vi "SS Class Init.vi"(7 "VI Refnum":refnum<vi>, 8 "error in (no error)":errorcluster, 9 "Init Data":variant, 10 "Device":string, 11 "Subsystem Class Temp Control in":refnum<class "Subsystem Class Temp Control.lvclass">) -> (0 "error out":errorcluster, 2 "Channel List":refnum<class "HK Item.lvclass">[](array[class]), 3 "Subsystem Class Temp Control out":refnum<class "Subsystem Class Temp Control.lvclass">)   [LabVIEW 2022 SP3, in "Subsystem Class Temp Control.lvclass"]
uses:
  Subsystem Class Temp Control.lvclass
  hk-channel-class/hk-channel-class/HK Item/HK Item.lvclass
  Subsystem Class.lvclass
  Subsystem Class Temp Control.lvclass/Subsystem Class Temp Control.ctl
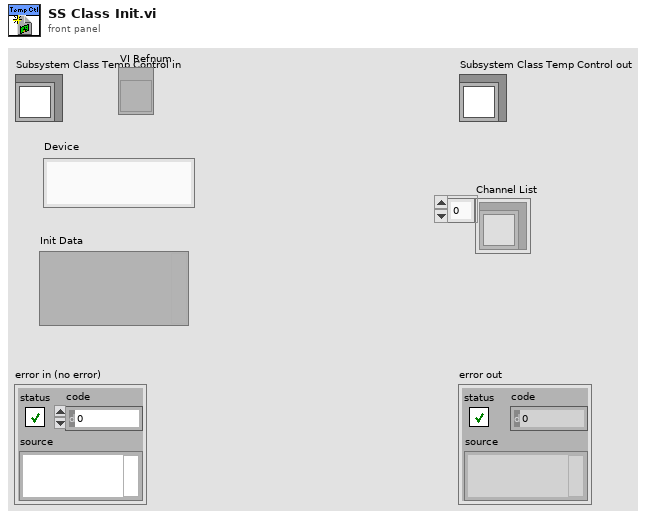
[diagram p1: front panel]
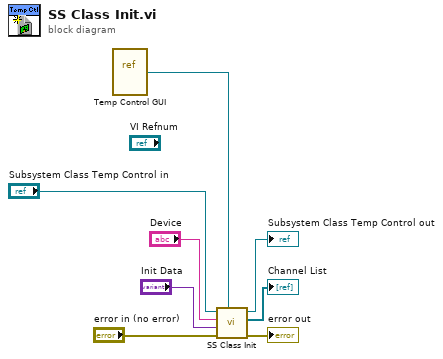
[diagram p0: block diagram]
diagram:
  n1 = vi-ref "Temp Control GUI.vi"() -> (w1:refnum<vi>)
  n2 = call-parent "SS Class Init.vi"("VI Refnum"=w1, "error in (no error)"="error in (no error)", "Init Data"="Init Data", "Device"="Device", "Subsystem Class in"="Subsystem Class Temp Control in") -> ("error out"=→"error out":errorcluster, "Channel List"=→"Channel List":refnum<class "HK Item.lvclass">[], "Subsystem Class out"=→"Subsystem Class Temp Control out":refnum<class "Subsystem Class Temp Control.lvclass">)  [unwired: 4 in]
